vi "OP600ZP_BDD.vi"(8 "errin":errorcluster, 11 "BDD":T1) -> (0 "error out":errorcluster)   [LabVIEW 2020]
panel:
  out "chaîne concaténée":string
  # "SCAN ____________________________"
  # "SEALING ____________________________"
  # "CONTI ____________________________"
  # "CAN BAT / VEH ____________________________"
  # "PARK ____________________________"
  # "ISO ____________________________"
  # "OCV ____________________________"
  # "CAPA ____________________________"
  # "PRECHARGE ____________________________"
  # "DCIR ____________________________"
  # "PARK 2  ____________________________"
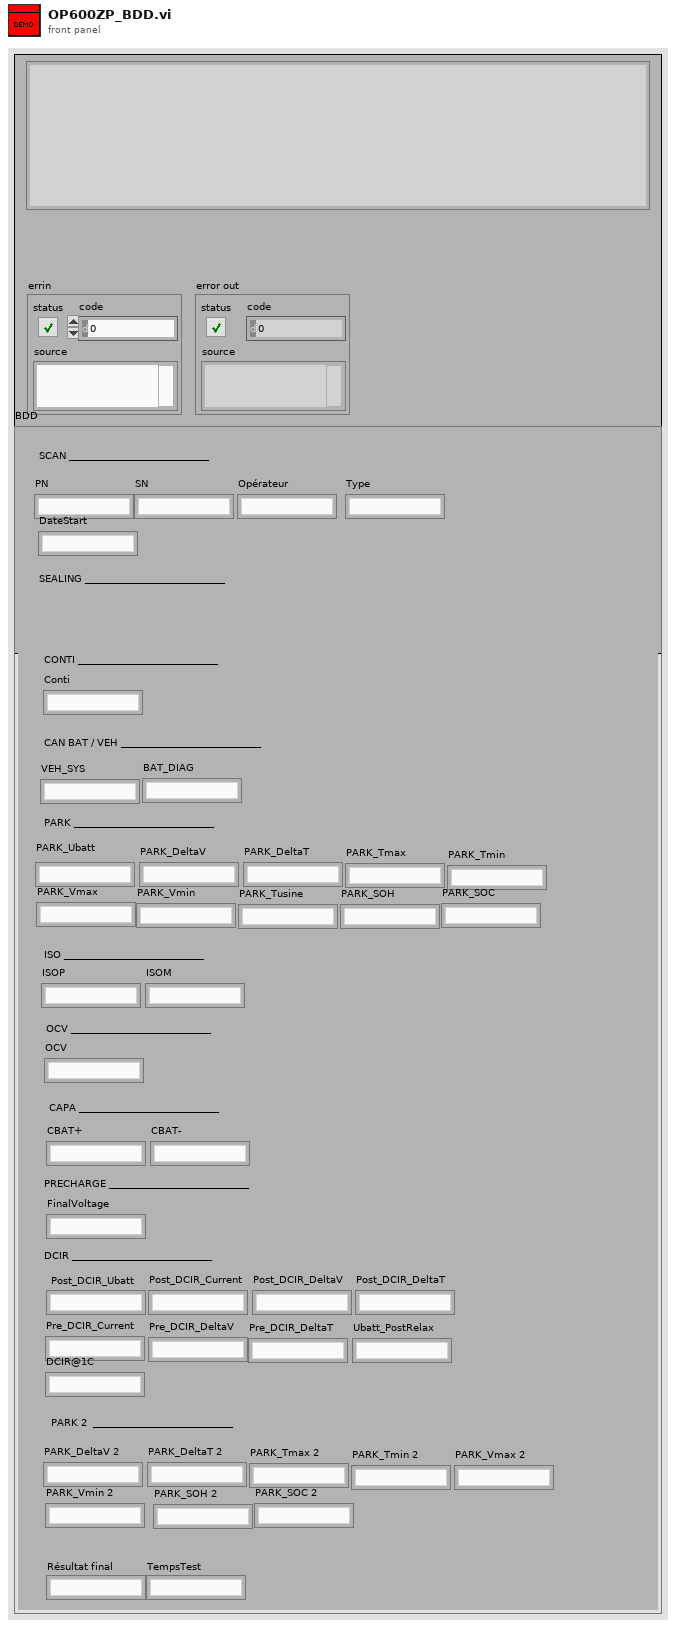
[diagram p1: front panel]
types:
  T1 = cluster{"PN":string, "SN":string, "Opérateur":string, "Type":string, "DateStart":string, "Conti":string, "VEH_SYS":string, "BAT_DIAG":string, "PARK_Ubatt":string, "PARK_DeltaV":string, "PARK_DeltaT":string, "PARK_Tmax":string, "PARK_Tmin":string, "PARK_Vmax":string, "PARK_Vmin":string, "PARK_Tusine":string, "PARK_SOH":string, "PARK_SOC":string, "ISOP":string, "ISOM":string, "OCV":string, "CBAT+":string, "CBAT-":string, "FinalVoltage":string, "Post_DCIR_Ubatt":string, "Post_DCIR_Current":string, "Post_DCIR_DeltaV":string, "Post_DCIR_DeltaT ":string, "Pre_DCIR_Current":string, "Pre_DCIR_DeltaV":string, "Pre_DCIR_DeltaT":string, "Ubatt_PostRelax":string, "DCIR@1C":string, "PARK_DeltaV 2":string, "PARK_DeltaT 2":string, "PARK_Tmin 2":string, "PARK_Tmax 2":string, "PARK_Vmax 2":string, "PARK_Vmin 2":string, "PARK_SOH 2":string, "PARK_SOC 2":string, "Résultat final":string, "TempsTest":string}
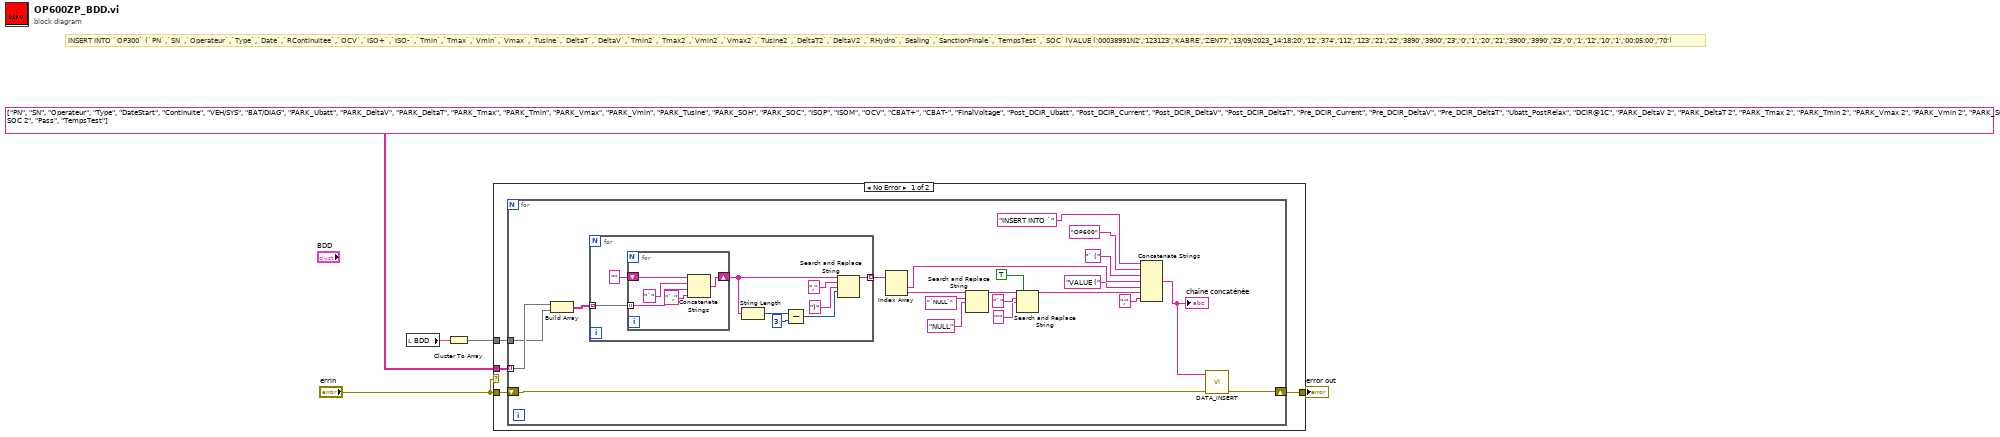
[diagram p0: block diagram]
diagram:
  # "INSERT INTO `OP300` (`PN`,`SN`,`Operateur`,`Type`,`Date`,`RContinuitee`,`OCV`,`ISO+`,`ISO-`,`Tmin`,`Tmax`,`Vmin`,`Vmax`,`Tusine`,`DeltaT`,`DeltaV`,`Tmin2`,`Tmax2`,`Vmin2`,`Vmax2`,`Tusine2`,`DeltaT2`,`DeltaV2`,`RHydro`,`Sealing`,`SanctionFinale`,`TempsTest`,`SOC`)VALUE ('00038991N2','123123','KABRE','ZEN77','13/09/2023_14:18:20','12','374','112','123','21','22','3890','3900','23','0','1','20','21','3900','3990','23','0','1','12','10','1','00:05:00','70')"
  n1 = local read "BDD"() -> (w1:T1)
  n2 = Cluster To Array(cluster=w1) -> (array=w2:string[])
  n3 = case shown="No Error" "errin" {
    tunnel: "errin" -> [w9 w45]
    tunnel: [w8 w45] -> w5
    tunnel: string[][] [["PN", "SN", "Operateur", "Type", "DateStart", "Continuite", "VEH/SYS", "BAT/DIAG", "PARK_Ubatt", "PARK_DeltaV", "PARK_DeltaT", "PARK_Tmax", "PARK_Tmin", "PARK_Vmax", "PARK_Vmin", "PARK_Tusine", "PARK_SOH", "PARK_SOC", "ISOP", "ISOM", "OCV", "CBAT+", "CBAT-", "FinalVoltage", "Post_DCIR_Ubatt", "Post_DCIR_Current", "Post_DCIR_DeltaV", "Post_DCIR_DeltaT", "Pre_DCIR_Current", "Pre_DCIR_DeltaV", "Pre_DCIR_DeltaT", "Ubatt_PostRelax", "DCIR@1C", "PARK_DeltaV 2", "PARK_DeltaT 2", "PARK_Tmax 2", "PARK_Tmin 2", "PARK_Vmax 2", "PARK_Vmin 2", "PARK_SOH 2", "PARK_SOC 2", "Pass", "TempsTest"]] -> [w7 _]
    tunnel: w2 -> [w6 _]
    frame No Error {
      n4 = for {
        shift-right: [w11] -> w8
        shift-left: w9 -> [w12]
        tunnel: w7 -> [w15] mode=indexing
        tunnel: w6 -> [w14]
        n5 = Build Array(w15, w14) -> (w30:string[][])
        n6 = for {
          tunnel: [w31] -> w16 mode=indexing
          tunnel: w30 -> [w39] mode=indexing
          n7 = for {
            shift-right: [w42] -> w32
            shift-left: "" -> [w41]
            tunnel: w39 -> [w40] mode=indexing
            n8 = Concatenate Strings(w41, "`" ("string"), w40, "`," ("string")) -> (w42:string)
          }
          n9 = String Length(string=w32) -> (length=w37:i32)
          n10 = Subtract(x=w37, y=3) -> (x-y=w35:i32)
          n11 = Search and Replace String(input string=w32, search string=",", replace string=")" ("replace string (\"\")"), offset=w35) -> (result string=w31:string)  [unwired: 4 in, 3 out]
        }
        n12 = Index Array(array=w16) -> (element #1=w26:string, element #2=w27:string)  [unwired: 2 in]
        n13 = Search and Replace String(input string=w27, search string="`NULL`", replace string="NULL" ("replace string (\"\")")) -> (result string=w28:string)  [unwired: 5 in, 3 out]
        n14 = Search and Replace String(replace all?=TRUE ("replace all? (F)"), input string=w28, search string="`", replace string="'" ("replace string (\"\")")) -> (result string=w29:string)  [unwired: 4 in, 3 out]
        n15 = Concatenate Strings("INSERT INTO `" ("string"), "OP600", "` (" ("string"), w26, "VALUE (" ("string"), w29, ";" ("string")) -> (w10:string)
        "chaîne concaténée" <- w10
        n16 = call <userlib>:"DATA_INSERT.vi"("errin"=w12, "INSERT"=w10) -> ("errout"=w11:errorcluster)  [unwired: 9 in]
      }
    }
    frame Error {
    }
  }
  "error out" <- w5
